vi "GetSize.vi"(8 "error in (no error)":errorcluster, 11 "reference in":refnum<class "Row.lvclass">) -> (0 "error out":errorcluster, 2 "Dimensions":T1, 3 "reference in":refnum<class "Row.lvclass">)   [LabVIEW 2012, in "Row.lvclass"]
uses:
  Row.lvclass
  Glyph_class/Dimensions.ctl
  Character_class/Character.lvclass
  Glyph_class/Glyph.lvclass
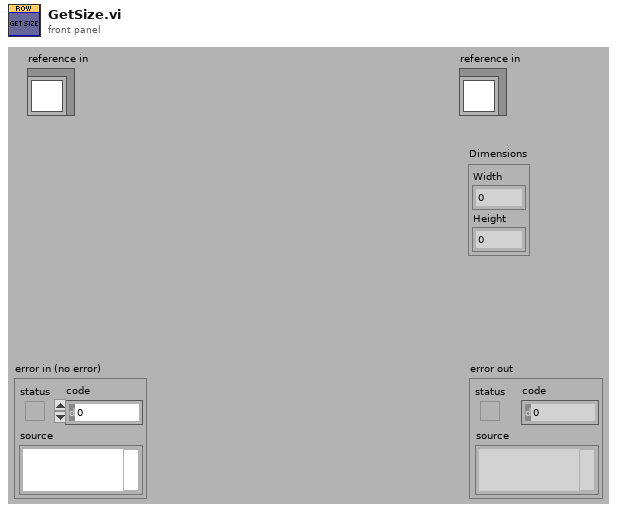
[diagram p1: front panel]
types:
  T1 = typedef "Glyph.lvclass/Dimensions.ctl" = cluster{"Width":i32, "Height":i32}
  T2 = typedef "Row.lvclass/ObjectAttributes.ctl" = cluster{"Characters":refnum<class "Character.lvclass">[], "StartPoint":T3, "CharacterSpacing":i32}
  T3 = typedef "Glyph.lvclass/Position.ctl" = cluster{"X":i32, "Y":i32}
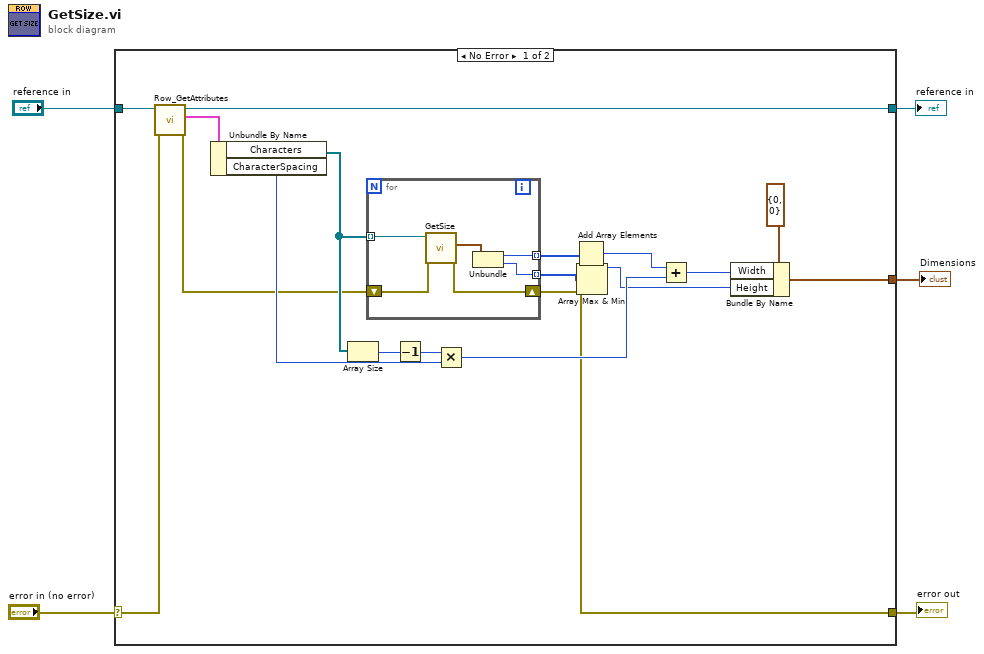
[diagram p0: block diagram]
diagram:
  n1 = case shown="No Error" "error in (no error)" {
    selector: "error in (no error)" -> [w23 w31]
    tunnel: [w8 w31] -> w4
    tunnel: [w20 w30] -> w2
    tunnel: "reference in" -> [w21 w30]
    tunnel: [w10 _] -> w1
    frame No Error {
      n2 = call "Row_GetAttributes.vi"("error in (no error)"=w23, "reference in"=w21) -> ("error out"=w9:errorcluster, "Data"=w22:T2, "reference out"=w20:refnum<class "Row.lvclass">)  [unwired: 6 in, 1 out]
      n3 = Unbundle By Name(w22) -> ("Characters"=w18:refnum<class "Character.lvclass">[], "CharacterSpacing"=w15:i32)
      n4 = Array Size(array=w18) -> (size(s)=w17:i32)
      n5 = for {
        tunnel: w18 -> [w29] mode=indexing
        tunnel: [w26] -> w19 mode=indexing
        tunnel: [w28] -> w7 mode=indexing
        shift-right: [w24] -> w8
        shift-left: w9 -> [w25]
        n6 = call-dynamic "GetSize.vi"("error in (no error)"=w25, "reference in"=w29) -> ("error out"=w24:errorcluster, "Dimensions"=w27:T1)  [unwired: 7 in, 1 out]
        n7 = Unbundle(w27) -> ("Width"=w26:i32, "Height"=w28:i32)
      }
      n8 = Decrement(x=w17) -> (x-1=w16:i32)
      n9 = Multiply(x=w16, y=w15) -> (x*y=w14:i32)
      n10 = Add Array Elements(numeric array=w19) -> (sum=w13:i32)
      n11 = Array Max & Min(array=w7) -> (max value=w6:i32)  [unwired: 3 out]
      n12 = Add(x=w13, y=w14) -> (x+y=w11:i32)
      n13 = Bundle By Name(cluster=T1 {"Width"=0, "Height"=0} ("Dimensions"), "Width"=w11, "Height"=w6) -> (w10:T1)
    }
    frame Error {
    }
  }
  "error out" <- w4
  "reference in" <- w2
  "Dimensions" <- w1
